vi "Config.vi"(8 "error in (no error)":errorcluster, 10 "Setting":T1={"Freq"=1000.0, "Range"=enum."10m Ohm", "Measurements"=enum."Impedence"} {"Freq" min=0.1 max=1050.0 step=0.01 format="%_5e"}, 11 "Hioki BT4560B in":refnum<class "Hioki BT4560B.lvclass">) -> (0 "error out":errorcluster, 3 "Hioki BT4560B out":refnum<class "Hioki BT4560B.lvclass">)   [LabVIEW 2021, in "Concrete.lvlib" / "Hioki BT4560B.lvclass"]
uses:
  Hioki BT4560B.lvclass
  Hioki BT4560B.lvclass/Hioki BT4560B.ctl
  <instrlib>/HIOKI BT4560/HIOKI BT4560.lvlib
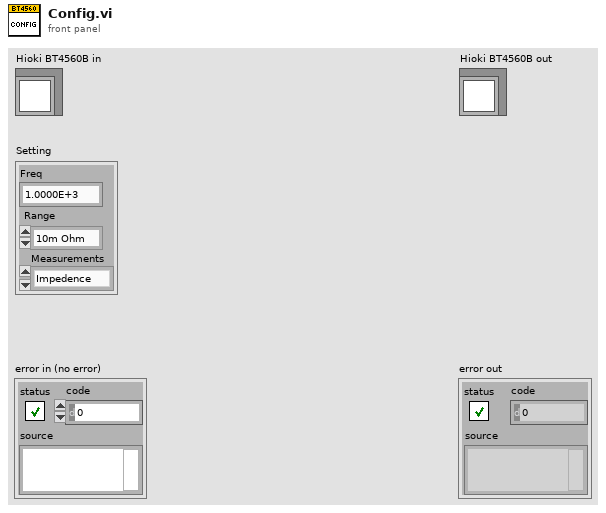
[diagram p1: front panel]
types:
  T1 = cluster{"Freq":dbl, "Range":enum16{"3m Ohm", "10m Ohm", "100m Ohm"}, "Measurements":enum16{"Impedence", "Phase Angle", "OCV"}}
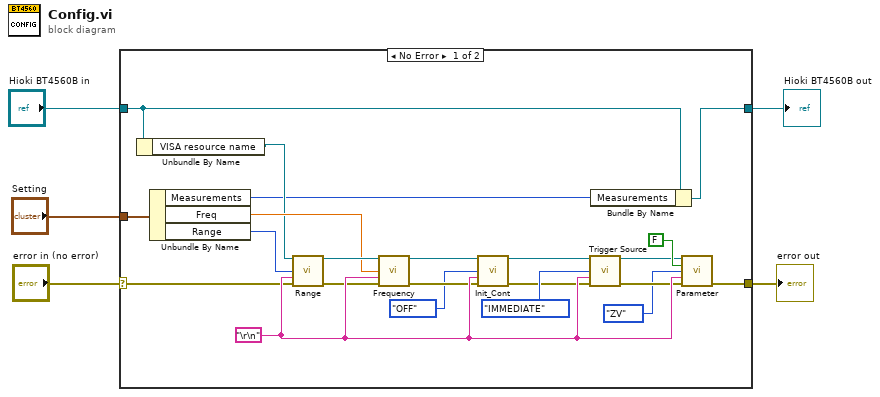
[diagram p0: block diagram]
diagram:
  n1 = case shown="No Error" "error in (no error)" {
    selector: "error in (no error)" -> [w14 w29]
    tunnel: [w13 w29] -> w4
    tunnel: [w7 w28] -> w2
    tunnel: "Hioki BT4560B in" -> [w8 w28]
    tunnel: "Setting" -> [w11 _]
    frame No Error {
      w26 = "\r\n" ("End of Line Constant")
      n2 = Unbundle By Name(w8) -> ("VISA resource name"=w12:refnum<visa-resource-name>)
      n3 = Unbundle By Name(w11) -> ("Measurements"=w6:enum16{"Impedence", "Phase Angle", "OCV"}, "Freq"=w15:dbl, "Range"=w10:enum16{"3m Ohm", "10m Ohm", "100m Ohm"})
      n4 = call <instrlib>:"Range.vi"("VISA session"=w12, "Range set"=w10, "Terminator"=w26, "error in (no error)"=w14) -> ("dup VISA session"=w16:refnum<visa-resource-name>, "error out"=w17:errorcluster)  [unwired: 8 in, 2 out]
      n5 = call <instrlib>:"Frequency.vi"("VISA session"=w16, "Freq set"=w15, "Terminator"=w26, "error in (no error)"=w17) -> ("dup VISA session"=w23:refnum<visa-resource-name>, "error out"=w22:errorcluster)  [unwired: 8 in, 2 out]
      n6 = call <instrlib>:"Init_Cont.vi"("VISA session"=w23, "Cont Meas set"=enum16{"OFF", "ON"}."OFF", "Terminator"=w26, "error in (no error)"=w22) -> ("dup VISA session"=w24:refnum<visa-resource-name>, "error out"=w18:errorcluster)  [unwired: 8 in, 2 out]
      n7 = call <instrlib>:"Trigger Source.vi"("VISA session"=w24, "Trigger Source set"=enum16{"EXTERNAL", "IMMEDIATE"}."IMMEDIATE", "Terminator"=w26, "error in (no error)"=w18) -> ("dup VISA session"=w25:refnum<visa-resource-name>, "error out"=w19:errorcluster)  [unwired: 8 in, 2 out]
      n8 = Bundle By Name(cluster=w8, "Measurements"=w6) -> (w7:refnum<class "Hioki BT4560B.lvclass">)
      n9 = call <instrlib>:"Parameter.vi"("VISA session"=w25, "Set/Query (F: Set)"=FALSE, "Parameter set"=enum16{"RV", "ZV", "R", "Z", "V"}."ZV", "Terminator"=w26, "error in (no error)"=w19) -> ("error out"=w13:errorcluster)  [unwired: 7 in, 3 out]
    }
    frame Error {
    }
  }
  "error out" <- w4
  "Hioki BT4560B out" <- w2
